vi "PH_Calorimeter_USB.PC Start.vi"(0 "i ref in":refnum<vi>, 5 "error in (no error)":errorcluster) -> (14 "i ref out":refnum<vi>, 19 "error out":errorcluster)   [LabVIEW 2014, in "PH_Calorimeter_USB.lvlib"]
doc: "This is the proc case \"Start\"."
uses:
  PH_Calorimeter_USB.lvlib
  PH_Common/PH_Common.lvlib
panel:
  in  "Cursor List":T1(array[cluster])=[{"Name"="x", "Color"=0, "Style"=0, "Point Style"=0, "Name Visible"=FALSE, "Allow Drag"=FALSE, "Lock Style"=0, "Plot"=0, "Index"=0, "Position"={"X"=0.0, "Y"=0.0}}]
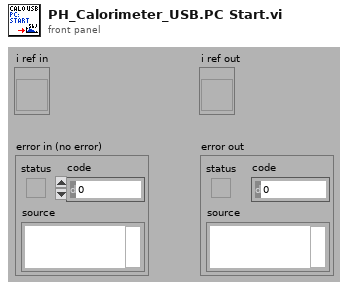
[diagram p1: front panel]
types:
  T1 = cluster{"Name":string, "Color":u32, "Style":u8, "Point Style":u8, "Name Visible":bool, "Allow Drag":bool, "Lock Style":u32, "Plot":u32, "Index":i32, "Position":cluster{"X":dbl, "Y":dbl}}[]
  T2 = typedef "PH_Calorimeter_USB.lvlib/PH_Calorimeter_USB.i attribute.ctl" = cluster{"GUI Refs":cluster{"Delete":refnum<vi>, "Start":refnum<vi>, "Energy":refnum<vi>, "Calorimeter":refnum<vi>, "Trigger":refnum<vi>, "Calo Calibration":refnum<vi>, "Time Base":refnum<vi>, "Device":refnum<vi>, "Graph Raw Data":refnum<vi>, "Graph Result":refnum<vi>}, "DAQ Instance":string, "Data":dbl[][], "Controller Instance":string, "Energy [J]":dbl, "Calorimeter":T3, "Trigger":T4, "Time Base":T5, "Calo Calibration":T6, "Serial Number":string}
  T3 = typedef "PH_Calorimeter_USB.lvlib/PH_Calorimeter_USB.Calorimeter Settings.ctl" = cluster{"Channel":tag, "Min Value [V]":dbl, "Max Value  [V]":dbl}
  T4 = typedef "PH_Calorimeter_USB.lvlib/PH_Calorimeter_USB.Trigger Settings.ctl" = cluster{"Channel":tag, "Min Value [V]":dbl, "Max Value  [V]":dbl, "Level [V]":dbl, "Wait Time [s]":dbl, "Length [Samples]":i32}
  T5 = typedef "PH_Calorimeter_USB.lvlib/PH_Calorimeter_USB.Time Base Settings.ctl" = cluster{"Samples per Channel":i32, "Rate [Hz]":i32}
  T6 = typedef "PH_Calorimeter_USB.lvlib/PH_Calorimeter_USB.Calorimeter Calibration Settings.ctl" = cluster{"T 1/e [s]":dbl, "Sensitivity  [Vs/J]":dbl}
  T7 = cluster{"Name":string, "Color":u32, "Style":u8, "Point Style":u8, "Name Visible":bool, "Allow Drag":bool, "Lock Style":u32, "Plot":u32, "Index":i32, "Position":cluster{"X":dbl, "Y":dbl}}
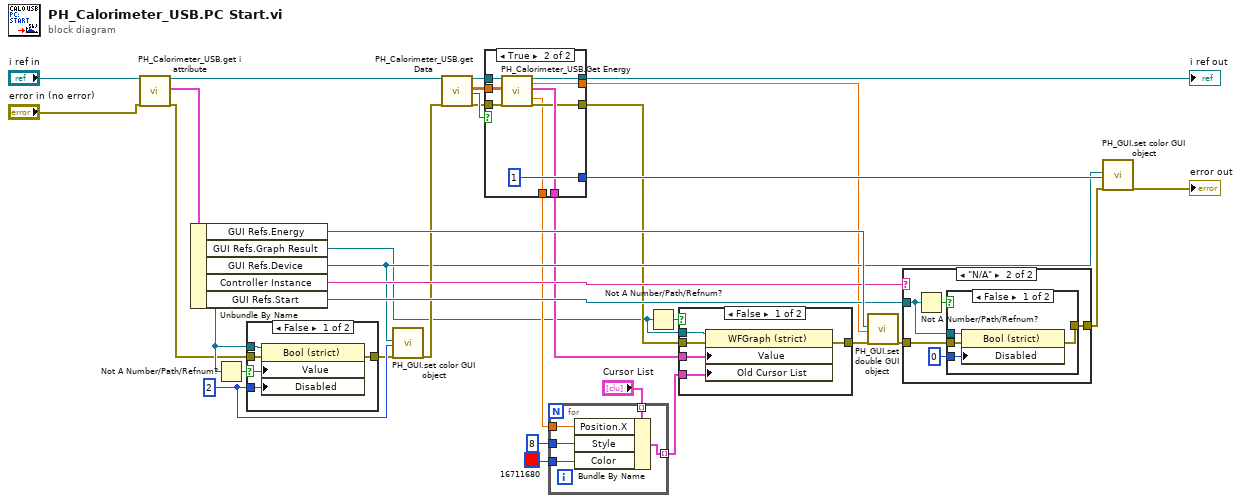
[diagram p0: block diagram]
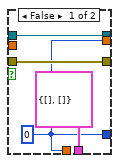
[diagram p5: hidden frame]
diagram:
  w27 = u8 2 ("Disabled")
  n1 = call "PH_Calorimeter_USB.get i attribute.vi"("i ref in"="i ref in", "error in (no error)"="error in (no error)") -> ("i ref out"=w18:refnum<vi>, "i attribute"=w20:T2, "error out"=w22:errorcluster)  [unwired: 15 in]
  n2 = Unbundle By Name(w20) -> ("GUI Refs.Energy"=w32:refnum<vi>, "GUI Refs.Graph Result"=w5:refnum<vi>, "GUI Refs.Device"=w14:refnum<vi>, "Controller Instance"=w30:string, "GUI Refs.Start"=w28:refnum<vi>)
  n3 = Not A Number/Path/Refnum?(number/path/refnum=w28) -> (NaN/Path/Refnum?=w21:bool)
  n4 = case shown="False" w21 {
    selector: w21 -> [w36 _]
    tunnel: w28 -> [w38 _]
    tunnel: w22 -> [w37 w39]
    tunnel: [w35 w39] -> w24
    tunnel: w27 -> [w34 _]
    frame False {
      n5 = property class="Bool (strict)"(reference=w38, error in=w37, "Value"=w36, "Disabled"=w34) -> (error out=w35:errorcluster)  [unwired: 1 out]
    }
    frame True {
    }
  }
  n6 = call "PH_GUI.set color GUI object.vi"("GUI object Ref"=w14, "State"=w27, "error in (no error)"=w24) -> ("error out"=w23:errorcluster)  [unwired: 16 in]
  n7 = call "PH_Calorimeter_USB.get Data.vi"("i ref in"=w18, "error in (no error)"=w23) -> ("i ref out"=w15:refnum<vi>, "raw data"=w3:dbl[][], "got Data"=w25:bool, "error out"=w16:errorcluster)  [unwired: 14 in]
  n8 = case shown="True" w25 {
    tunnel: [w43 w47] -> w2
    tunnel: w15 -> [w43 w51]
    tunnel: [w42 w46] -> w13
    tunnel: w16 -> [w42 w50]
    tunnel: [w40 1 ("State")] -> w29
    tunnel: [w40 w49] -> w4
    tunnel: [cluster{dbl[], dbl[]} {[], []} ("Graph") w48] -> w11
    tunnel: [w40 w45] -> w6
    tunnel: w3 -> [_ w44]
    frame False {
      w40 = 0 ("State")
    }
    frame True {
      n9 = call "PH_Calorimeter_USB.Get Energy.vi"("i ref in"=w51, "Raw Data"=w44, "error in (no error)"=w50) -> ("i ref out"=w47:refnum<vi>, "Energy [J]"=w49:dbl, "Graph"=w48:cluster{dbl[], dbl[]}, "Offset Time [s]"=w45:dbl, "error out"=w46:errorcluster)  [unwired: 12 in]
    }
  }
  "i ref out" <- w2
  n10 = for {
    tunnel: "Cursor List" -> [w57] mode=indexing
    tunnel: [w56] -> w7 mode=indexing
    tunnel: w6 -> [w55]
    tunnel: u8 8 ("Style") -> [w54]
    tunnel: u32 16711680 ("Color Box") -> [w53]
    n11 = Bundle By Name(cluster=w57, "Position.X"=w55, "Style"=w54, "Color"=w53) -> (w56:T7)
  }
  n12 = Not A Number/Path/Refnum?(number/path/refnum=w5) -> (NaN/Path/Refnum?=w33:bool)
  n13 = case shown="False" w33 {
    tunnel: w5 -> [w62 _]
    tunnel: w13 -> [w61 w63]
    tunnel: [w60 w63] -> w12
    tunnel: w11 -> [w59 _]
    tunnel: w7 -> [w58 _]
    frame False {
      n14 = property class="WFGraph (strict)"(reference=w62, error in=w61, "Value"=w59, "Old Cursor List"=w58) -> (error out=w60:errorcluster)  [unwired: 1 out]
    }
    frame True {
    }
  }
  n15 = call "PH_GUI.set double GUI object.vi"("GUI object Ref"=w32, "value"=w4, "error in (no error)"=w12) -> ("error out"=w31:errorcluster)  [unwired: 16 in]
  n16 = case shown="\"N/A\"" w30 {
    tunnel: [w64 w68] -> w26
    tunnel: w31 -> [w64 w66]
    tunnel: w28 -> [_ w65]
    frame "False", Default {
    }
    frame "N/A" {
      n17 = Not A Number/Path/Refnum?(number/path/refnum=w65) -> (NaN/Path/Refnum?=w69:bool)
      n18 = case shown="False" w69 {
        tunnel: w65 -> [w73 _]
        tunnel: w66 -> [w72 w74]
        tunnel: [w71 w74] -> w68
        tunnel: u8 0 ("Disabled") -> [w70 _]
        frame False {
          n19 = property class="Bool (strict)"(reference=w73, error in=w72, "Disabled"=w70) -> (error out=w71:errorcluster)  [unwired: 1 out]
        }
        frame True {
        }
      }
    }
  }
  n20 = call "PH_GUI.set color GUI object.vi"("GUI object Ref"=w14, "State"=w29, "error in (no error)"=w26) -> ("error out"=→"error out":errorcluster)  [unwired: 16 in]
